vi "ProtoSnap_RB.vi"() -> ()   [LabVIEW 2012]
uses:
  <userlib>/BotSpeak/VIs/Direct/BotSpeak_Control.ctl
panel:
  in  "Bot Settings":T1
  out "List":string[](array[string])
  out "page":u8
  in  "Intro Help":bool
  in  "Previous":bool
  in  "Next":bool
  in  "Stop Button":bool
  in  "Pages":T2(tab)
  in  "Test Button":bool
  in  "Com Port":u16(ring) items=["ASRL7  (/dev/cu.usbserial-AM01VFXW)"]
  in  "Hardware":u16(ring) items=["Arduino Uno", "BeagleBone Serial", "BeagleBone", "Console Only", "EV3", "EvalRIO", "Launchpad", "PICAXE 80M", "Raspberry Pi", "Thymio"]
  out "firmware":dbl
  out "Light":u8(slide) scale=0.0..100.0
  in  "Open LED":bool
  in  "LED":cluster{"Red":bool, "Green":bool, "Blue":bool}
  in  "Open":bool
  in  "Port":u8=13
  in  "State":enum16{"LO", "HI"}(ring)
  in  "Run":bool
  # "Getting Started\n\nThe goal of this book is to get you started in LabVIEW with the Protosnap - you will need 1 protosnap - please connect it up."
  # "Test BotSpeak\n\nThe next step is to test it out.  Choose your hardware and port (if you have not plugged your Protosnap in yet, plug it in and select Arduino Uno).  Push REFRESH to text the connection and see if you get Firmware 0.9 back."
  # "Test the ProtoSnap\n\nTry pushing the button or reading the light sensor.  You can click on any of the areas to see the program that is running"
  # "Writing LabVIEW Code\n\nPush the Run button - does the light go off?  Change it from LO to HI - and run it again.  What happens? Try changing the Port - from pin 13 to some other number.  This is called a LabVIEW diagram - it is where your program resides - this program is simple - it changes the state of pin 13.  Click on the Open button to open a slightly more complicated program."
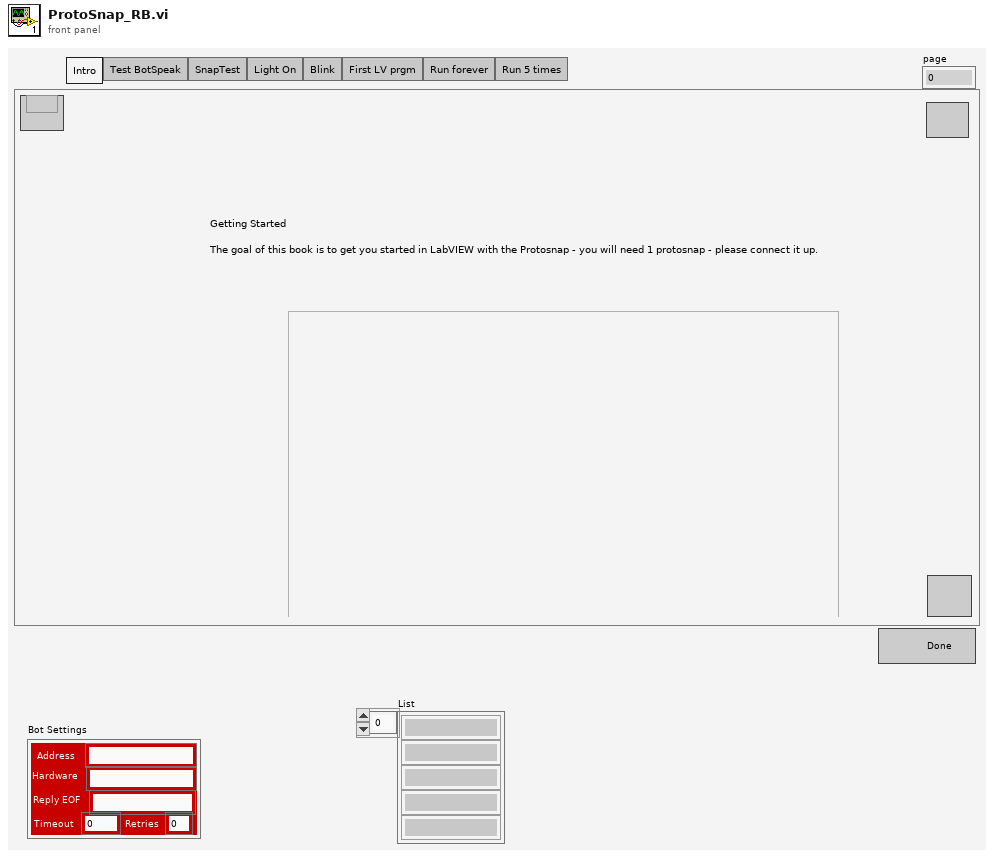
[diagram p1: front panel]
types:
  T1 = typedef "BotSpeak_Control.ctl" = cluster{"Address":string, "Reply EOF":string, "Hardware":string, "Retries":i8, "Timeout":i32}
  T2 = enum32{"Intro", "Test BotSpeak", "SnapTest", "Light On", "Blink", "First LV prgm", "Run forever", "Run 5 times"}
  T3 = typedef "BotSpeak.HardwareSpecs.ctl" = cluster{"Hardware Name":string, "Hardware URL":string, "ComType":enum16{"Undefined", "Serial", "TCPIP", "Console", "EV3"}, "TCP Port":i32, "DefaultAddress":string, "Retries":i32, "Translate":enum16{"None", "Tiny", "URAPI"}, "MaxScriptSize":i32, "MaxVarNumber":i32, "StartupWait":i32, "Patience":i32, "Startup Patience":i32, "Hardware Help":string, "Com Protocol":string, "Translator":cluster{"BotSpeak CMD":string, "CMD out":string}[], "Init Code":string, "Variable Format":enum16{"INT", "FLOAT", "FIXED"}}
  T4 = enum16{"Undefined", "Serial", "TCPIP", "Console", "EV3"}
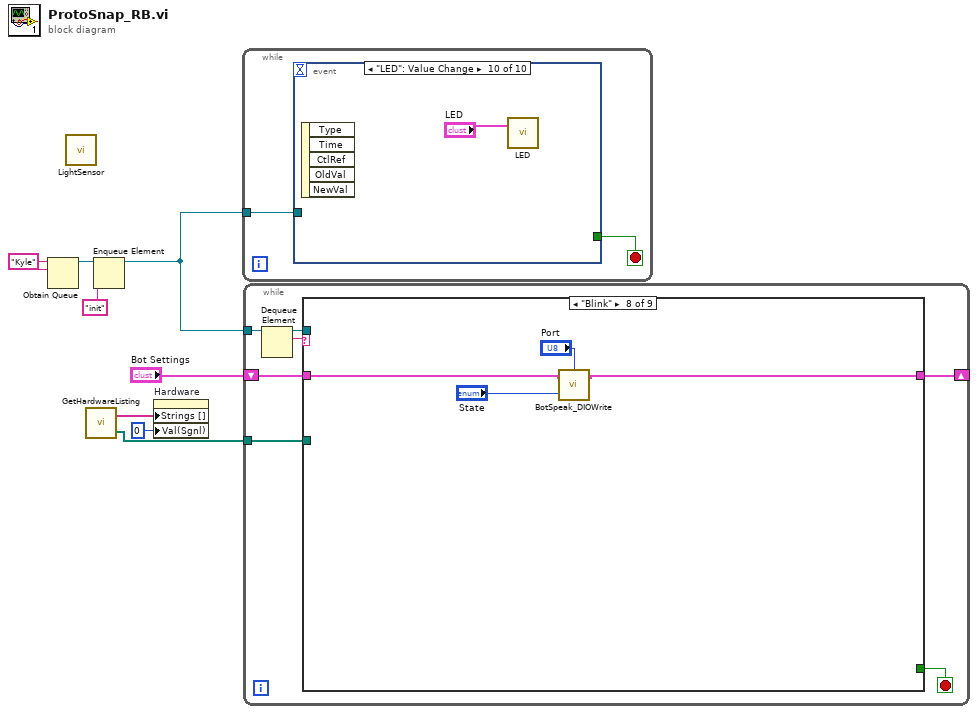
[diagram p0: block diagram]
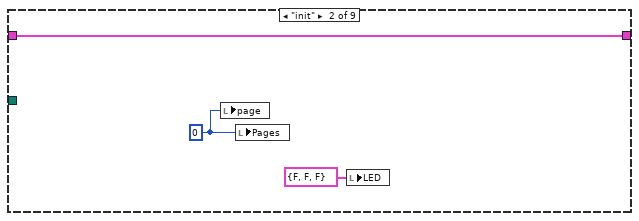
[diagram p3: hidden frame]
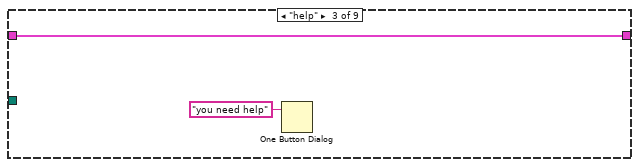
[diagram p4: hidden frame]
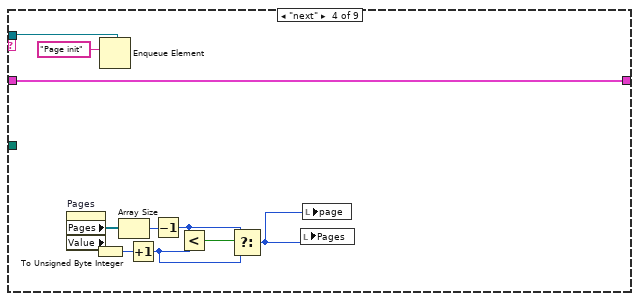
[diagram p5: hidden frame]
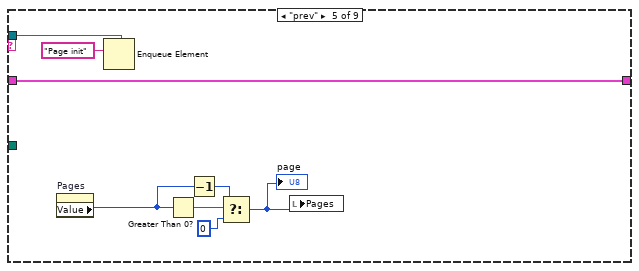
[diagram p6: hidden frame]
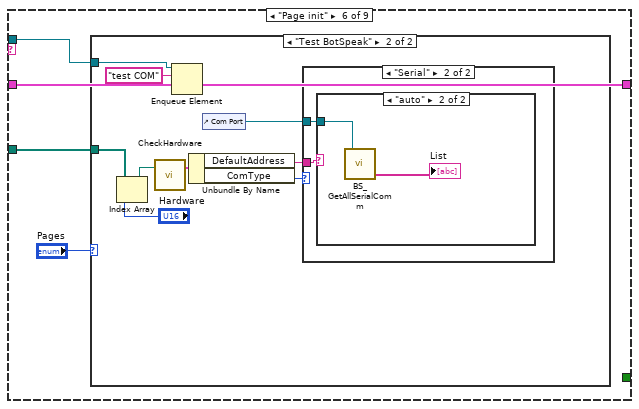
[diagram p7: hidden frame]
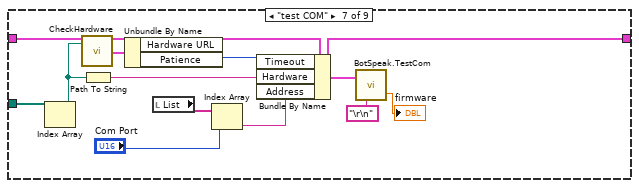
[diagram p11: hidden frame]
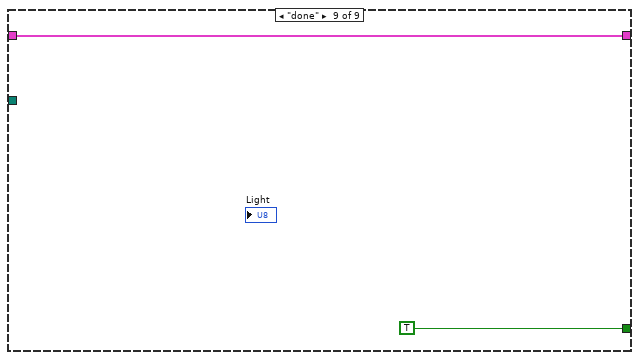
[diagram p12: hidden frame]
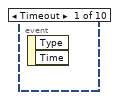
[diagram p13: hidden frame]
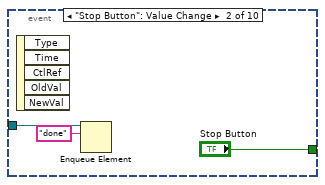
[diagram p14: hidden frame]
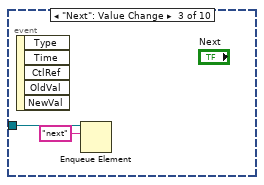
[diagram p15: hidden frame]
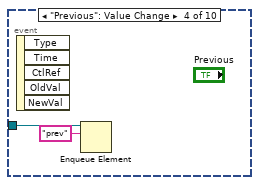
[diagram p16: hidden frame]
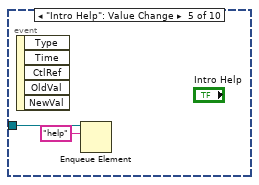
[diagram p17: hidden frame]
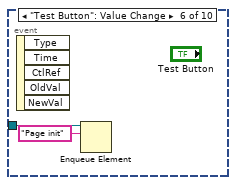
[diagram p18: hidden frame]
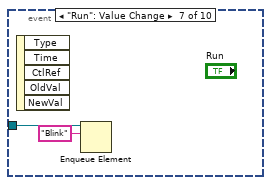
[diagram p19: hidden frame]
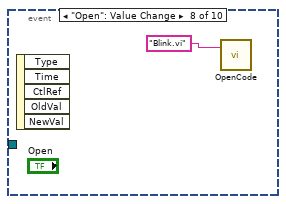
[diagram p20: hidden frame]
diagram:
  w7 = "Kyle" ("name (unnamed)")
  n1 = Obtain Queue(name (unnamed)=w7, element data type=w7) -> (queue out=w8:refnum<queue>)  [unwired: 3 in, 2 out]
  n2 = call "LightSensor.vi"() -> ()  [unwired: 12 in]
  n3 = call <userlib>:"GetHardwareListing.vi"() -> ("Devices"=w2:path[], "Array"=w4:string[])  [unwired: 2 in]
  n4 = Enqueue Element(queue=w8, element="init") -> (queue out=w6:refnum<queue>)  [unwired: 2 in, 2 out]
  n5 = property on="Hardware" class="Ring (strict)"("Strings []"=w4, "Val(Sgnl)"=u16 0 ("Value (Signaling)")) -> ()  [unwired: 2 in, 2 out]
  n6 = while {
    tunnel: w6 -> [w9]
    stop <- w10 stop-if-true
    n7 = event shown="[9] \"LED\": Value Change" {
      selector: _ -> [_ _ _ _ _ _ _ _ _ _]
      dyn-events: _ -> [_ _ _ _ _ _ _ _ _ _]
      timeout: _ -> [_ _ _ _ _ _ _ _ _ _]
      tunnel: [_ "Stop Button" _ _ _ _ _ _ _ _] -> w10
      tunnel: w9 -> [_ w12 w15 w17 w19 w21 w23 _ _ _]
      event Timeout {
        n8 = event-data() -> ()  [unwired: 1 in, 2 out]
      }
      event "Stop Button": Value Change {
        n9 = event-data() -> ()  [unwired: 1 in, 5 out]
        n10 = Enqueue Element(queue=w12, element="done") -> ()  [unwired: 2 in, 3 out]
      }
      event "Next": Value Change {
        n11 = event-data() -> ()  [unwired: 1 in, 5 out]
        n12 = Enqueue Element(queue=w15, element="next") -> ()  [unwired: 2 in, 3 out]
      }
      event "Previous": Value Change {
        n13 = event-data() -> ()  [unwired: 1 in, 5 out]
        n14 = Enqueue Element(queue=w17, element="prev") -> ()  [unwired: 2 in, 3 out]
      }
      event "Intro Help": Value Change {
        n15 = event-data() -> ()  [unwired: 1 in, 5 out]
        n16 = Enqueue Element(queue=w19, element="help") -> ()  [unwired: 2 in, 3 out]
      }
      event "Test Button": Value Change {
        n17 = event-data() -> ()  [unwired: 1 in, 5 out]
        n18 = Enqueue Element(queue=w21, element="Page init") -> ()  [unwired: 2 in, 3 out]
      }
      event "Run": Value Change {
        n19 = event-data() -> ()  [unwired: 1 in, 5 out]
        n20 = Enqueue Element(queue=w23, element="Blink") -> ()  [unwired: 2 in, 3 out]
      }
      event "Open": Value Change {
        n21 = event-data() -> ()  [unwired: 1 in, 5 out]
        n22 = call "OpenCode.vi"("Code name"="Blink.vi" ("name or relative path")) -> ()  [unwired: 3 in]
      }
      event "Open LED": Value Change {
        n23 = event-data() -> ()  [unwired: 1 in, 5 out]
        n24 = call "OpenCode.vi"("Code name"="LED.vi" ("name or relative path")) -> ()  [unwired: 3 in]
      }
      event "LED": Value Change {
        n25 = event-data() -> ()  [unwired: 1 in, 5 out]
        n26 = call "LED.vi"("LED"="LED") -> ()  [unwired: 3 in]
      }
    }
  }
  n27 = while {
    tunnel: w6 -> [w33]
    tunnel: w2 -> [w29]
    shift-right: [w27] -> _
    shift-left: "Bot Settings" -> [w28]
    stop <- w31 stop-if-true
    n28 = Dequeue Element(queue=w33) -> (queue out=w30:refnum<queue>, element=w32:string)  [unwired: 2 in, 2 out]
    n29 = case shown="\"Blink\"" w32 {
      tunnel: [_ _ _ _ _ _ _ _ TRUE] -> w31
      tunnel: w30 -> [_ _ _ w41 w52 w59 _ _ _]
      tunnel: w29 -> [_ _ _ _ _ w61 w80 _ _]
      tunnel: w28 -> [w34 w36 w38 w40 w51 w60 w78 w89 w92]
      tunnel: [w34 w36 w38 w40 w51 w60 w76 w88 w92] -> w27
      frame Default {
      }
      frame "init" {
        w37 = 0
        n30 = local write "page"(w37) -> ()
        n31 = local write "Pages"(w37) -> ()
        n32 = local write "LED"(cluster{"Red":bool, "Green":bool, "Blue":bool} {"Red"=FALSE, "Green"=FALSE, "Blue"=FALSE} ("LED")) -> ()
      }
      frame "help" {
        n33 = One Button Dialog(message="you need help") -> ()  [unwired: 1 in, 1 out]
      }
      frame "next" {
        n34 = property on="Pages" class="TabCtl (strict)"() -> ("Pages"=w50:refnum<vi>[], "Value"=w47:T2)  [unwired: 2 in, 2 out]
        n35 = To Unsigned Byte Integer(number=w47) -> (unsigned 8bit integer=w44:u8)
        n36 = Enqueue Element(queue=w41, element="Page init") -> ()  [unwired: 2 in, 3 out]
        n37 = Array Size(array=w50) -> (size(s)=w48:i32)
        n38 = Increment(x=w44) -> (x+1=w46:u8)
        n39 = Decrement(x=w48) -> (x-1=w45:i32)
        n40 = Less?(x=w45, y=w46) -> (x < y?=w49:bool)
        n41 = Select(t=w45, s=w49, f=w46) -> (s? t:f=w43:i32)
        n42 = local write "Pages"(w43) -> ()
        n43 = local write "page"(w43) -> ()
      }
      frame "prev" {
        n44 = property on="Pages" class="TabCtl (strict)"() -> ("Value"=w55:T2)  [unwired: 2 in, 2 out]
        n45 = Enqueue Element(queue=w52, element="Page init") -> ()  [unwired: 2 in, 3 out]
        n46 = Greater Than 0?(x=w55) -> (x > 0?=w58:bool)
        n47 = Decrement(x=w55) -> (x-1=w54:T2)
        n48 = Select(t=w54, s=w58, f=0) -> (s? t:f=w56:u32)
        "page" <- w56
        n49 = local write "Pages"(w56) -> ()
      }
      frame "Page init" {
        n50 = case shown="\"Test BotSpeak\"" "Pages" {
          tunnel: w61 -> [_ w67]
          tunnel: w59 -> [_ w63]
          frame "Intro", Default {
          }
          frame "Test BotSpeak" {
            n51 = Index Array(array=w67, index="Hardware") -> (element=w68:path)
            n52 = call <userlib>:"CheckHardware.vi"("Hardware"=w68) -> ("HardwareSpecs"=w69:T3)  [unwired: 2 in]
            n53 = Enqueue Element(queue=w63, element="test COM") -> ()  [unwired: 2 in, 3 out]
            n54 = Unbundle By Name(w69) -> ("DefaultAddress"=w71:string, "ComType"=w70:T4)
            n55 = control-ref of="Com Port"() -> (w65:refnum<vi>)
            n56 = case shown="\"Serial\"" w70 {
              tunnel: w71 -> [_ w73]
              tunnel: w65 -> [_ w72]
              frame Default {
              }
              frame "Serial" {
                n57 = case shown="\"auto\"" w73 {
                  tunnel: w72 -> [_ w75]
                  frame Default {
                  }
                  frame "auto" {
                    n58 = call <userlib>:"BS_GetAllSerialComm.vi"("reference"=w75) -> ("List"=→"List":string[])  [unwired: 1 in, 2 out]
                  }
                }
              }
            }
          }
        }
      }
      frame "test COM" {
        n59 = Index Array(array=w80) -> (element=w83:path)  [unwired: 1 in]
        n60 = call <userlib>:"CheckHardware.vi"("Hardware"=w83) -> ("HardwareSpecs"=w82:T3)  [unwired: 2 in]
        n61 = Path To String(path=w83) -> (string=w85:string)
        n62 = Unbundle By Name(w82) -> ("Patience"=w84:i32)  [unwired: 1 out]
        n63 = local read "List"() -> (w81:string[])
        n64 = Index Array(array=w81, index="Com Port") -> (element=w77:string)
        n65 = Bundle By Name(cluster=w78, "Timeout"=w84, "Hardware"=w85, "Address"=w77) -> (w76:T1)
        n66 = call <userlib>:"BotSpeak.TestCom.vi"("Termination"="\r\n", "Bot Settings"=w76) -> ("firmware"=→"firmware":dbl)  [unwired: 1 out]
      }
      frame "Blink" {
        n67 = call <userlib>:"BotSpeak_DIOWrite.vi"("State"="State", "Bot Settings"=w89, "DIO Line"="Port") -> ("Bot Settings"=w88:T1)  [unwired: 1 out]
      }
      frame "done" {
      }
    }
  }
